vi "Kinesis - KDC101 - Connect.vi"() -> ()   [LabVIEW 2024]
doc: "Shows how to Start a motor control."
uses:
  C:/Users/goods/OneDrive/Desktop/Work/program/MOVER/Thorlabs.MotionControl.Controls.dll
  OneDrive/Desktop/Work/program/MOVER/Thorlabs.MotionControl.Controls.dll
panel:
  in  "Serial Number":string
  in  "?":bool
  in  "KCubeDCServoControl":refnum<k24>(container)
  # "Notes:"
  # "- Ensure that the appropriate .DLLs are copied into your Project Folder. Check that the correct bit type are used depending on your version of LabVIEW\ni.e. 32-bit or 64-bit.\n\n\n\n\n\n\n\n\n\n\n\n\n\n\n- Open the example VI through the LabVIEW Project Explorer to correctly load the User Interface from Thorlabs.MotionControl.Controls.dll."
  # "Thorlabs Hardware: KDC101 - K-Cube Brushed DC Servo Motor Controller\nhttps://www.thorlabs.com/newgrouppage9.cfm?objectgroup_id=2419\n\nDescription: This VI shows you how to initialize communication with and then disconnect from KDC101, in order to control DC Brushed Stages & Actuators.\n\nInstructions: \n1) Connect your KBD101 device to your PC & power the device, ensuring your stage/actutator is connected. For full device setup, the device product manual can be found on our website here. - https://www.thorlabs.com/thorproduct.cfm?partnumber=KDC101\n2) Enter the device serial number below.\n3) Click 'Run' in the LabVIEW Toolbar.\n4) To End the program, click the 'STOP' button."
  # "Example Image of .NET Controller - VI opened via Project Explorer/ not opened via Project Explorer"
  # "VI Not Opened via Project Explorer"
  # "VI Opened via Project Explorer"
  # "- To explore the range of methods available, please visit the .NET API, included with your Kinesis software.\n\n- For tips on building your own VIs with Thorlabs Motion Control Hardware, please see our LabVIEW Guide here.\nhttps://www.thorlabs.com/newgrouppage9.cfm?objectgroup_id=10285"
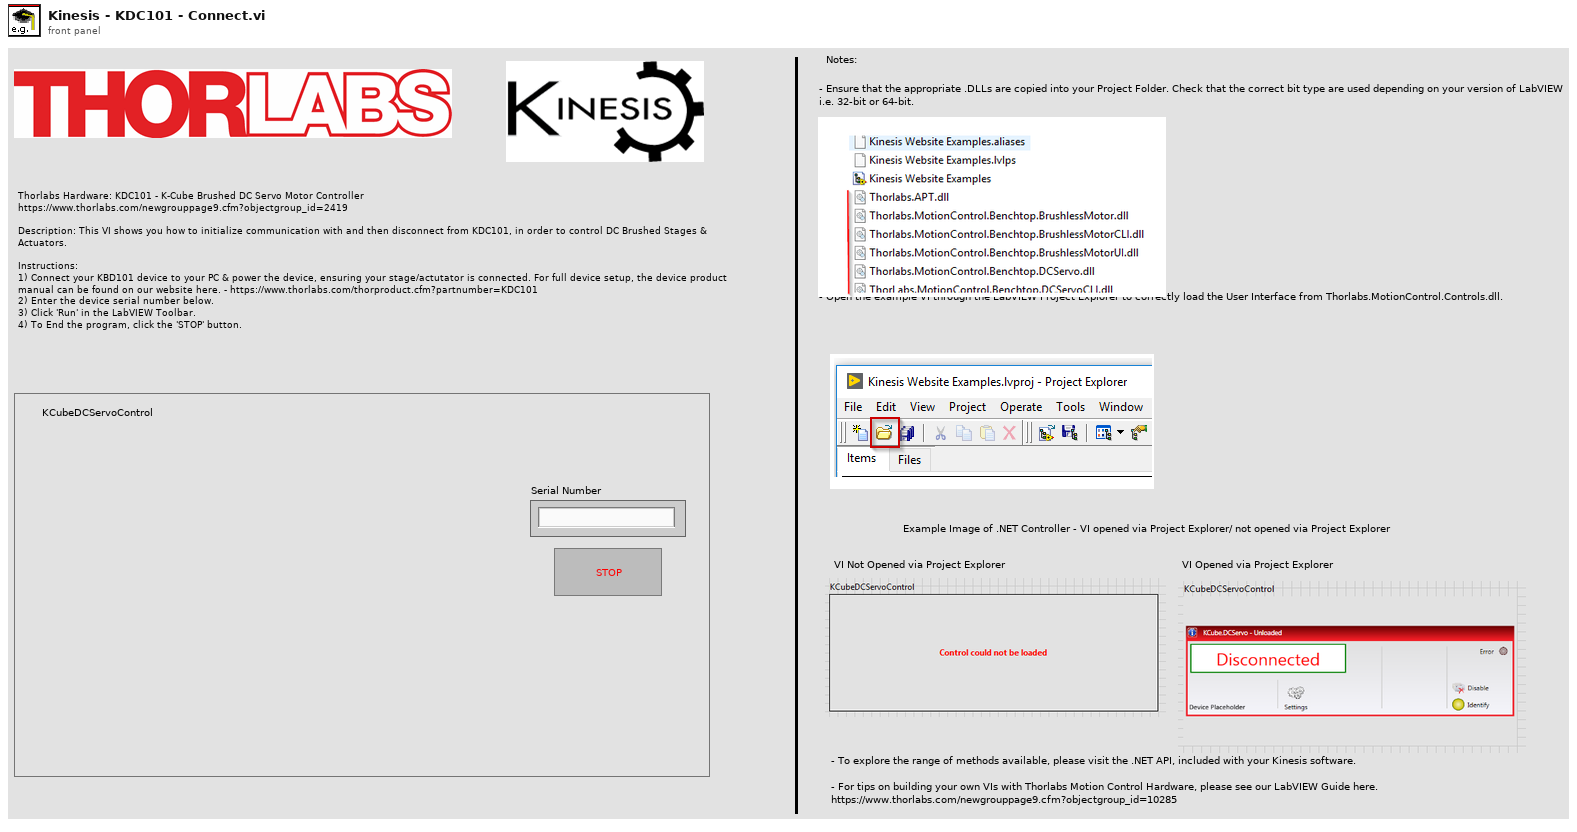
[diagram p1: front panel]
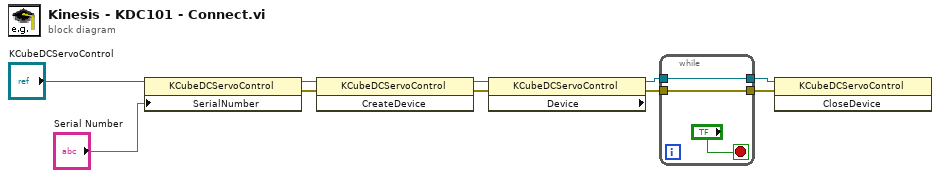
[diagram p0: block diagram]
diagram:
  n1 = property class="KCubeDCServoControl"(reference="KCubeDCServoControl", "SerialNumber"="Serial Number") -> (reference out=w9:refnum<k24>, error out=w6:errorcluster)  [unwired: 1 in]
  n2 = invoke class="KCubeDCServoControl" method="CreateDevice"(reference=w9, error in=w6) -> (reference out=w8:refnum<k24>, error out=w5:errorcluster)  [unwired: 1 in, 1 out]
  n3 = property class="KCubeDCServoControl" props=["Device"](reference=w8, error in=w5) -> (reference out=w2:refnum<k24>, error out=w4:errorcluster)  [unwired: 1 out]
  n4 = while {
    tunnel: [w12] -> w3
    tunnel: w4 -> [w12]
    tunnel: [w11] -> w1
    tunnel: w2 -> [w11]
    stop <- "?" stop-if-true
  }
  n5 = invoke class="KCubeDCServoControl" method="CloseDevice"(reference=w1, error in=w3) -> ()  [unwired: 1 in, 3 out]
